vi "CGI Datasheet Retrieve Channel Results.vi"(8 "error in (no error)":errorcluster, 10 "All Combined Fields":T1[](array[typedef]), 11 "Grouped Results":cluster{"Result Group":T9[]}[](array[cluster])) -> (0 "error out":errorcluster, 1 "First Item Run":string, 2 "First Item Path":string, 3 "Data Tree":T4[][](array[typedef]), 4 "First Item Test Type":string)   [LabVIEW 2011]
uses:
  TDMS/TDMS Model Number.ctl
  TDMS/TDMS Serial Number.ctl
  TDMS/TDMS File.ctl
  TDMS/TDMS Run.ctl
  TDMS/TDMS Channel (Sxx).ctl
  database/Fields/Field Record.ctl
  database/Fields/Field DataTypes.ctl
  database/Fields/Field NextItem.ctl
  www/cgi-bin/_cgi-lib/TDM_INDEX Record.ctl
panel:
  out "sum":u32
  out "time":u32
  out "Query result":T4[](array[typedef])
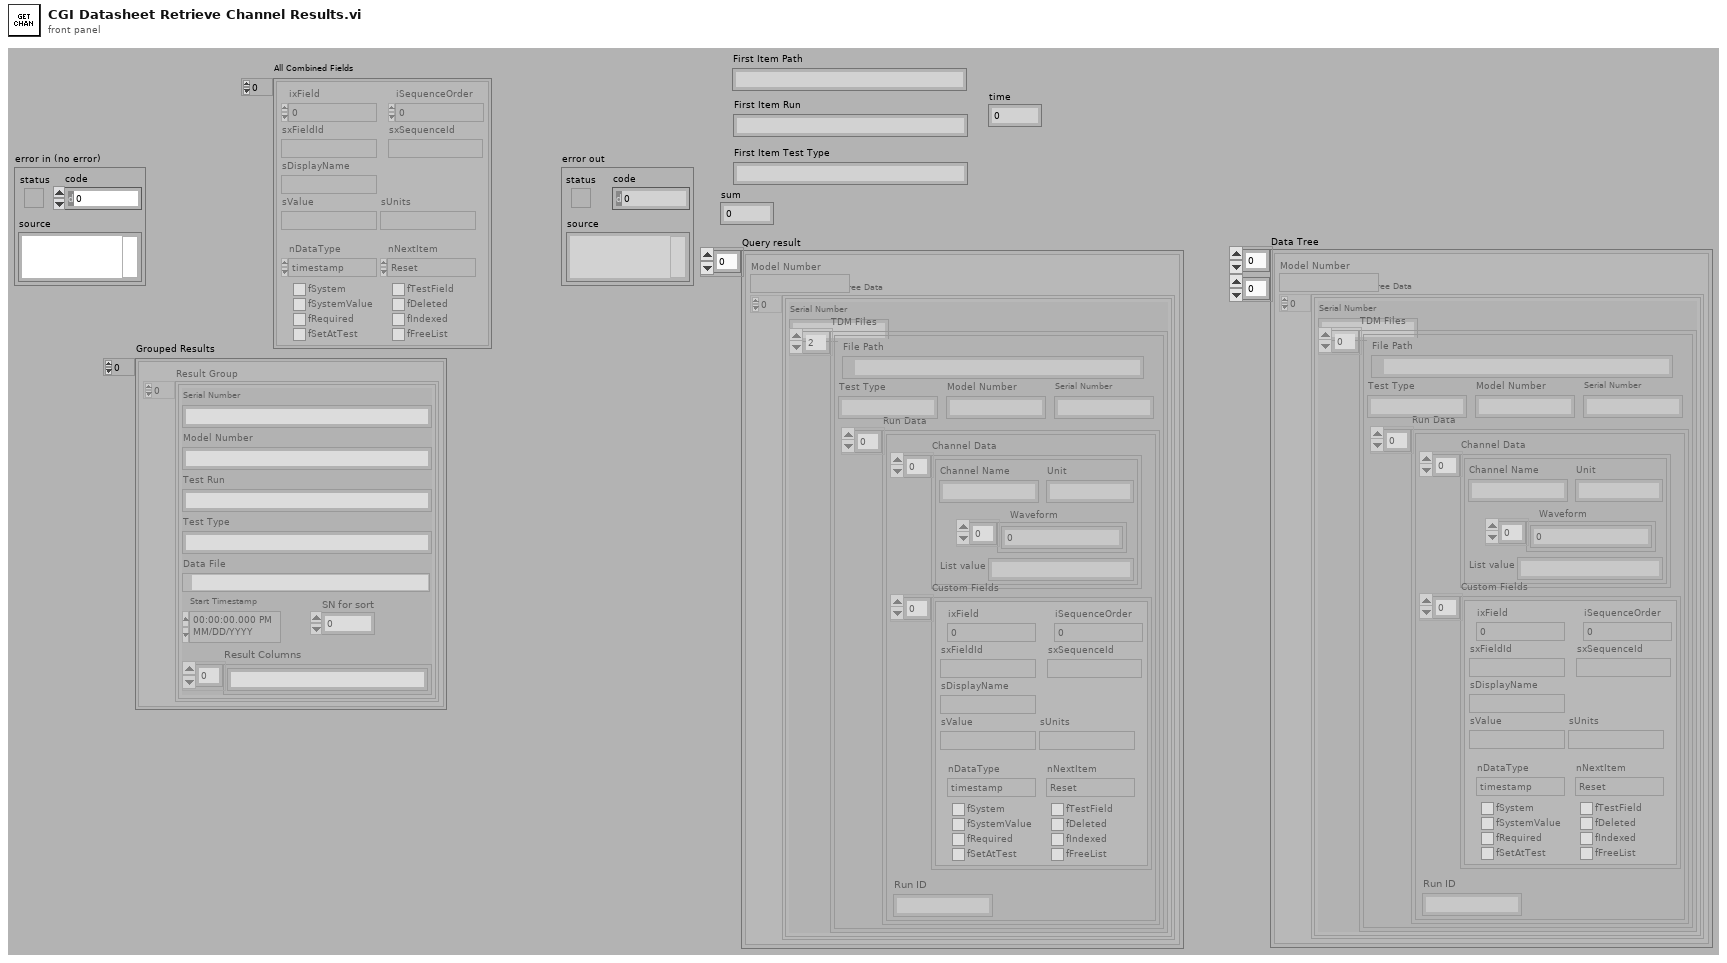
[diagram p1: front panel]
types:
  T1 = typedef "Field Record.ctl" = cluster{"ixField":i32, "iSequenceOrder":i32, "sxFieldId":string, "sxSequenceId":string, "sDisplayName":string, "sValue":string, "sUnits":string, "nDataType":T2, "nNextItem":T3, "fSystem":bool, "fSystemValue":bool, "fRequired":bool, "fSetAtTest":bool, "fTestField":bool, "fDeleted":bool, "fIndexed":bool, "fFreeList":bool}
  T2 = typedef "Field DataTypes.ctl" = enum32{"text", "numeric", "list", "timestamp", "boolean"}
  T3 = typedef "Field NextItem.ctl" = enum32{"Reset", "Retain", "Auto-Increment"}
  T4 = typedef "TDMS Model Number.ctl" = cluster{"Model Number":string, "Serial Number Tree Data":T5[]}
  T5 = typedef "TDMS Serial Number.ctl" = cluster{"Serial Number":string, "TDM Files":T6[]}
  T6 = typedef "TDMS File.ctl" = cluster{"File Path":path, "Run Data":T7[], "Serial Number":string, "Model Number":string, "Test Type":string}
  T7 = typedef "TDMS Run.ctl" = cluster{"Channel Data":T8[], "Custom Fields":T1[], "Run ID":string}
  T8 = typedef "TDMS Channel (Sxx).ctl" = cluster{"Channel Name":string, "Waveform":dbl[], "Unit":string, "List value":string}
  T9 = typedef "TDM_INDEX Record.ctl" = cluster{"Model Number":string, "SN for sort":i32, "Test Type":string, "Test Run":string, "Serial Number":string, "Start Timestamp":timestamp, "Data File":path, "Result Columns":string[]}
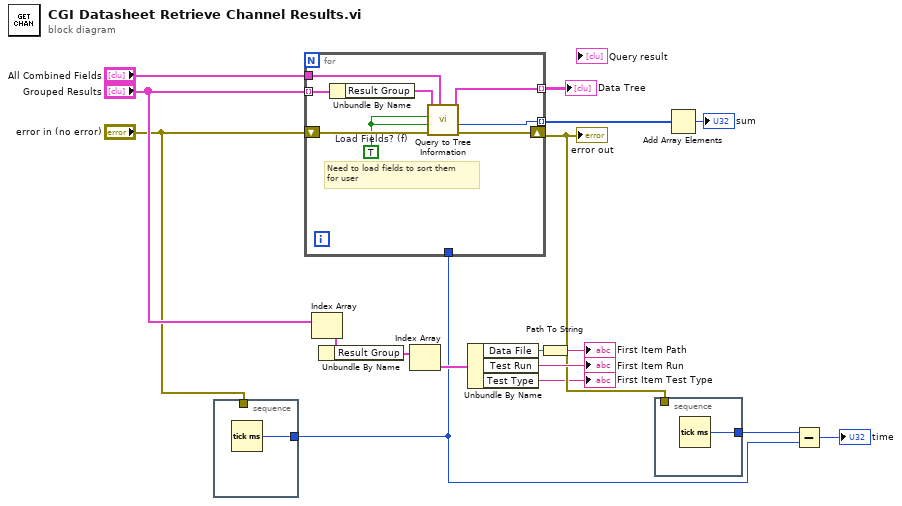
[diagram p0: block diagram]
diagram:
  n1 = stacked-sequence {
    tunnel: [w18] -> w5
    tunnel: "error in (no error)" -> [_]
    frame #0 {
      n2 = Tick Count (ms)() -> (millisecond timer value=w18:u32)
    }
  }
  n3 = for {
    shift-right: [w26] -> w9
    shift-left: "error in (no error)" -> [w23]
    tunnel: "Grouped Results" -> [w25] mode=indexing
    tunnel: [w21] -> w8 mode=indexing
    tunnel: [w20] -> w7 mode=indexing
    tunnel: w5 -> [_]
    tunnel: "All Combined Fields" -> [w19]
    w22 = TRUE  # Load Fields? (f)
    # "Need to load fields to sort them\nfor user"
    n4 = Unbundle By Name(w25) -> ("Result Group"=w24:T9[])
    n5 = call "Query to Tree Information.vi"("System or ALL Combined Fields"=w19, "error in (no error)"=w23, "Load data? (t)"=w22, "Load Fields? (f)"=w22, "Run Array"=w24) -> ("error out"=w26:errorcluster, "Total ms"=w20:u32, "Data Tree"=w21:T4[])  [unwired: 4 out]
  }
  "error out" <- w9
  "Data Tree" <- w8
  n6 = Index Array(array="Grouped Results") -> (element=w16:cluster{"Result Group":T9[]})  [unwired: 1 in]
  n7 = Unbundle By Name(w16) -> ("Result Group"=w15:T9[])
  n8 = Index Array(array=w15) -> (element=w14:T9)  [unwired: 1 in]
  n9 = Unbundle By Name(w14) -> ("Data File"=w13:path, "Test Run"=→"First Item Run":string, "Test Type"=→"First Item Test Type":string)
  n10 = Path To String(path=w13) -> (string=→"First Item Path":string)
  n11 = stacked-sequence {
    tunnel: [w27] -> w10
    tunnel: w9 -> [_]
    frame #0 {
      n12 = Tick Count (ms)() -> (millisecond timer value=w27:u32)
    }
  }
  n13 = Add Array Elements(numeric array=w7) -> (sum=→"sum":u32)
  n14 = Subtract(x=w10, y=w5) -> (x-y=→"time":u32)
